vi "Serial simulator.vi"() -> ()   [LabVIEW 2016]
panel:
  out "Array":i32[][](array[numeric])
  in  "stop":bool
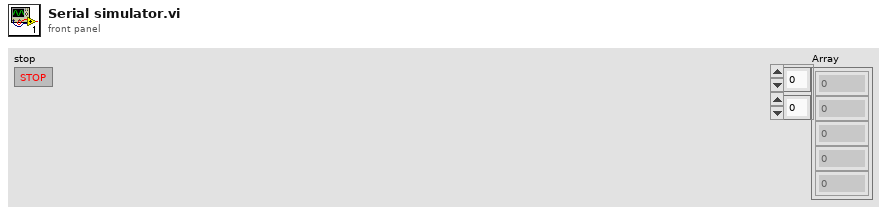
[diagram p1: front panel]
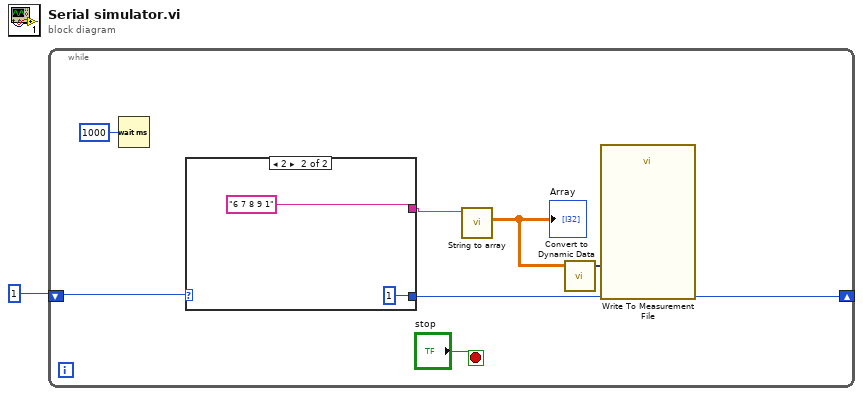
[diagram p0: block diagram]
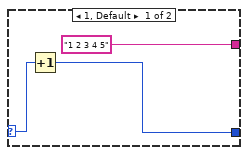
[diagram p2: hidden frame]
diagram:
  n1 = while {
    shift-right: [w7] -> _
    shift-left: 1 -> [w8]
    stop <- "stop" stop-if-true
    n2 = Wait (ms)(milliseconds to wait=u32 1000) -> ()  [unwired: 1 out]
    n3 = case shown="2" w8 {
      selector: w8 -> [w10 _]
      tunnel: ["1 2 3 4 5" "6 7 8 9 1"] -> w4
      tunnel: [w9 1] -> w7
      frame 1, Default {
        n4 = Increment(x=w10) -> (x+1=w9:i32)
      }
      frame 2 {
      }
    }
    n5 = call "String to array.vi"("String"=w4) -> ("Array"=w3:dbl[][])  [unwired: 10 in]
    "Array" <- w3
    n6 = call "Convert to Dynamic Data"("2D Array"=w3) -> ("Dynamic Data Type"=w2:dynamicdata)  [unwired: 3 in]
    n7 = call "Write To Measurement File"("Signals"=w2) -> ()  [unwired: 16 in, 3 out]
  }
